vi "Copy Image.vi"(1 "Image In":T1(plugin-control), 2 "Name":string) -> (0 "Image Out":T1(plugin-control))   [LabVIEW 2016]
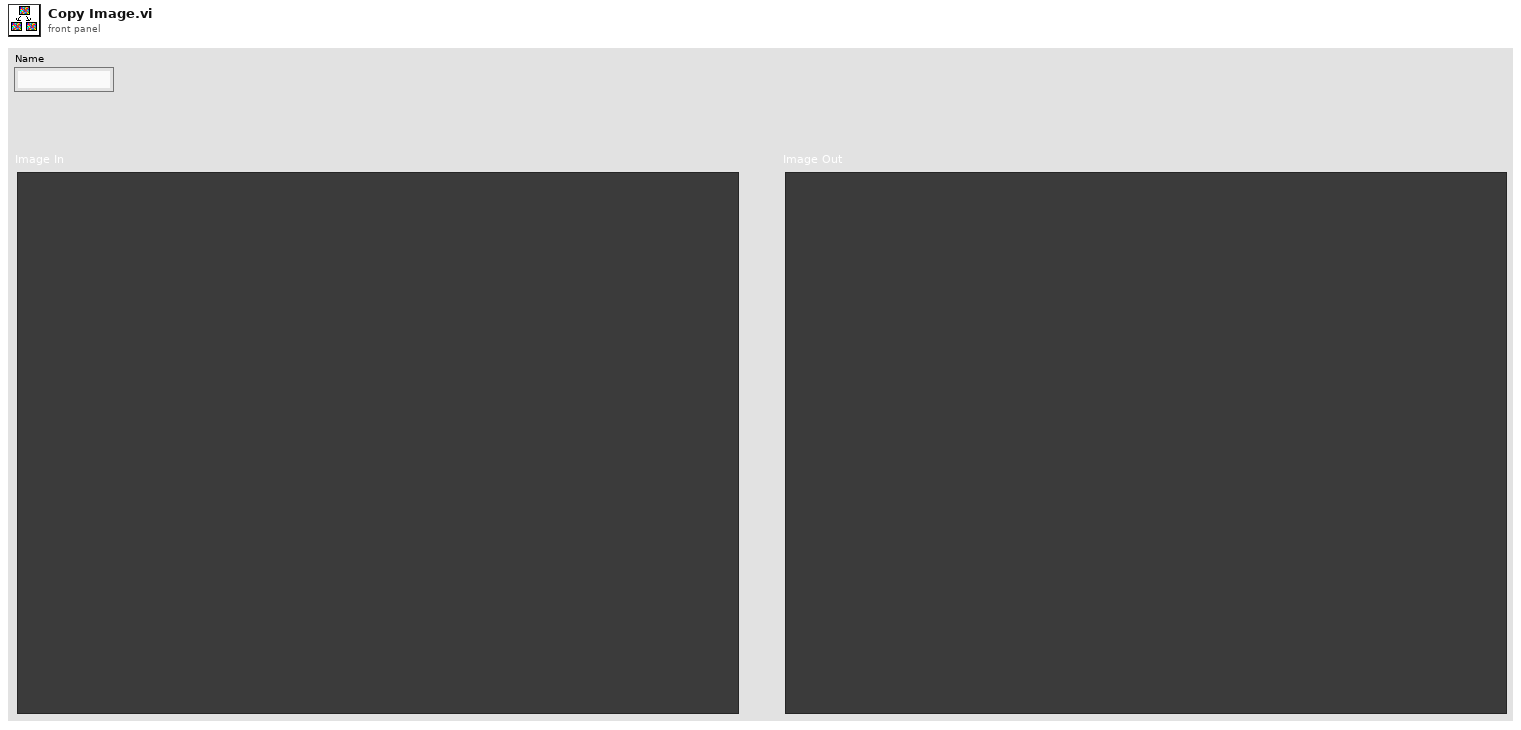
[diagram p1: front panel]
types:
  T1 = typedef "IMAQ Image.ctl" = refnum<image>
  T2 = typedef "Image Type" = u32
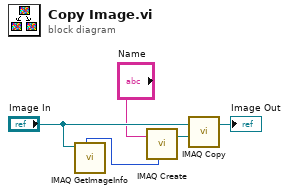
[diagram p0: block diagram]
diagram:
  n1 = call "IMAQ GetImageInfo"("Image"="Image In") -> ("Image Type"=w2:T2)  [unwired: 3 in, 7 out]
  n2 = call "IMAQ Create"("Image Name"="Name", "Image Type"=w2) -> ("New Image"=w4:T1)  [unwired: 3 in, 1 out]
  n3 = call "IMAQ Copy"("Image Dst"=w4, "Image Src"="Image In") -> ("Image Dst Out"=→"Image Out":T1)  [unwired: 4 in, 1 out]
